vi "Convert_Message_For_Signal_Processing.vi"(1 "String":string) -> (0 "Array":i16[](array[numeric]))   [LabVIEW 2024]
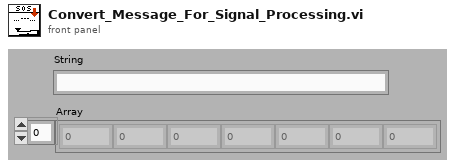
[diagram p1: front panel]
types:
  T1 = cluster{"0":bool[], "2":bool[], "4":bool[], "5":bool[], "6":bool[], "8":bool[], "9":bool[], "B":bool[], "C":bool[], "A":bool[], "D":bool[], "E":bool[], "7":bool[], "3":bool[], "1":bool[], "F":bool[], "G":bool[], "H":bool[], "I":bool[], "J":bool[], "K":bool[], "L":bool[], "M":bool[], "N":bool[], "O":bool[], "P":bool[], "Q":bool[], "R":bool[], "S":bool[], "T":bool[], "U":bool[], "V":bool[], "W":bool[], "X":bool[], "Y":bool[], "Z":bool[], ".":bool[], "?":bool[], ",":bool[], "/":bool[], "Space":bool[], "Null":bool[]}
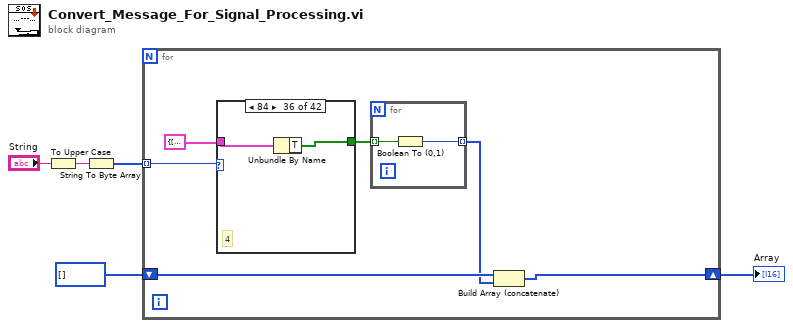
[diagram p0: block diagram]
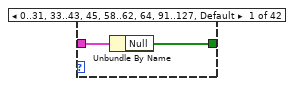
[diagram p2: hidden frame]
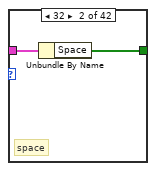
[diagram p3: hidden frame]
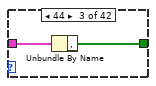
[diagram p4: hidden frame]
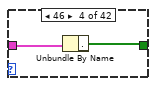
[diagram p5: hidden frame]
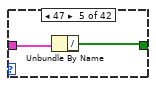
[diagram p6: hidden frame]
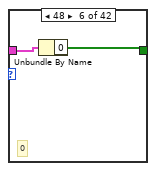
[diagram p7: hidden frame]
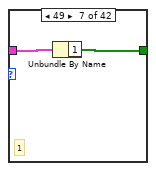
[diagram p8: hidden frame]
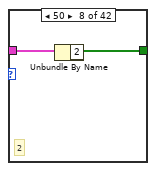
[diagram p9: hidden frame]
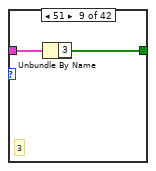
[diagram p10: hidden frame]
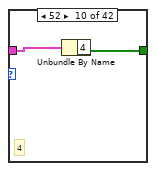
[diagram p11: hidden frame]
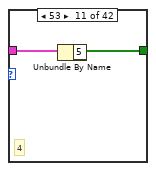
[diagram p12: hidden frame]
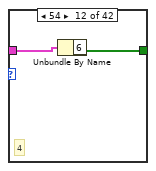
[diagram p13: hidden frame]
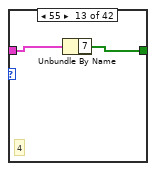
[diagram p14: hidden frame]
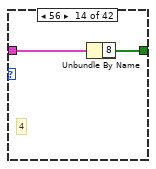
[diagram p15: hidden frame]
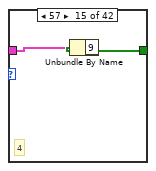
[diagram p16: hidden frame]
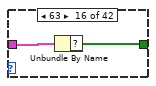
[diagram p17: hidden frame]
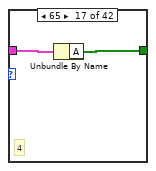
[diagram p18: hidden frame]
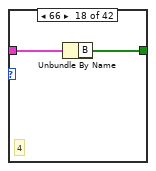
[diagram p19: hidden frame]
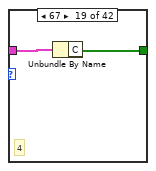
[diagram p20: hidden frame]
diagram:
  n1 = To Upper Case(1:"String") -> (0:w3:string)
  n2 = String To Byte Array(string=w3) -> (unsigned byte array=w4:u8[])
  n3 = for {
    tunnel: w4 -> [w10] mode=indexing
    shift-right: [w11] -> w1
    shift-left: i16[] [] -> [w9]
    n4 = case shown="84" w10 {
      tunnel: [w15 w17 w18 w20 w22 w25 w27 w29 w31 w33 w35 w37 w39 w41 w43 w45 w47 w49 w51 w53 w55 w57 w59 w61 w63 w65 w67 w69 w71 w73 w75 w77 w79 w81 w83 w85 w87 w89 w91 w92 w95 w97] -> w7
      tunnel: T1 {"0"=[TRUE, TRUE, TRUE, FALSE, TRUE, TRUE, TRUE, FALSE, TRUE, TRUE, TRUE, FALSE, TRUE, TRUE, TRUE, FALSE, TRUE, TRUE, TRUE, FALSE, FALSE, FALSE, FALSE, FALSE], "2"=[TRUE, FALSE, TRUE, FALSE, TRUE, TRUE, TRUE, FALSE, TRUE, TRUE, TRUE, FALSE, TRUE, TRUE, TRUE, FALSE, FALSE, FALSE, FALSE, FALSE], "4"=[TRUE, FALSE, TRUE, FALSE, TRUE, FALSE, TRUE, FALSE, TRUE, TRUE, TRUE, FALSE, FALSE, FALSE, FALSE, FALSE], "5"=[TRUE, FALSE, TRUE, FALSE, TRUE, FALSE, TRUE, FALSE, TRUE, FALSE, FALSE, FALSE, FALSE, FALSE], "6"=[TRUE, TRUE, TRUE, FALSE, TRUE, FALSE, TRUE, FALSE, TRUE, FALSE, TRUE, FALSE, FALSE, FALSE, FALSE, FALSE], "8"=[TRUE, TRUE, TRUE, FALSE, TRUE, TRUE, TRUE, FALSE, TRUE, TRUE, TRUE, FALSE, TRUE, FALSE, TRUE, FALSE, FALSE, FALSE, FALSE, FALSE], "9"=[TRUE, TRUE, TRUE, FALSE, TRUE, TRUE, TRUE, FALSE, TRUE, TRUE, TRUE, FALSE, TRUE, TRUE, TRUE, FALSE, TRUE, FALSE, FALSE, FALSE, FALSE, FALSE], "B"=[TRUE, TRUE, TRUE, FALSE, TRUE, FALSE, TRUE, FALSE, TRUE, FALSE, FALSE, FALSE, FALSE, FALSE], "C"=[TRUE, TRUE, TRUE, FALSE, TRUE, FALSE, TRUE, TRUE, TRUE, FALSE, TRUE, FALSE, FALSE, FALSE, FALSE, FALSE], "A"=[TRUE, FALSE, TRUE, TRUE, TRUE, FALSE, FALSE, FALSE, FALSE, FALSE], "D"=[TRUE, TRUE, TRUE, FALSE, TRUE, FALSE, TRUE, FALSE, FALSE, FALSE, FALSE, FALSE], "E"=[TRUE, FALSE, FALSE, FALSE, FALSE, FALSE], "7"=[TRUE, TRUE, TRUE, FALSE, TRUE, TRUE, TRUE, FALSE, TRUE, FALSE, TRUE, FALSE, TRUE, FALSE, FALSE, FALSE, FALSE, FALSE], "3"=[TRUE, FALSE, TRUE, FALSE, TRUE, FALSE, TRUE, TRUE, TRUE, FALSE, TRUE, TRUE, TRUE, FALSE, FALSE, FALSE, FALSE, FALSE], "1"=[TRUE, FALSE, TRUE, TRUE, TRUE, FALSE, TRUE, TRUE, TRUE, FALSE, TRUE, TRUE, TRUE, FALSE, TRUE, TRUE, TRUE, FALSE, FALSE, FALSE, FALSE, FALSE], "F"=[TRUE, FALSE, TRUE, FALSE, TRUE, TRUE, TRUE, FALSE, TRUE, FALSE, FALSE, FALSE, FALSE, FALSE], "G"=[TRUE, TRUE, TRUE, FALSE, TRUE, TRUE, TRUE, FALSE, TRUE, FALSE, FALSE, FALSE, FALSE, FALSE], "H"=[TRUE, FALSE, TRUE, FALSE, TRUE, FALSE, TRUE, FALSE, FALSE, FALSE, FALSE, FALSE], "I"=[TRUE, FALSE, TRUE, FALSE, FALSE, FALSE, FALSE, FALSE], "J"=[TRUE, FALSE, TRUE, TRUE, TRUE, FALSE, TRUE, TRUE, TRUE, FALSE, TRUE, TRUE, TRUE, FALSE, FALSE, FALSE, FALSE, FALSE], "K"=[TRUE, TRUE, TRUE, FALSE, TRUE, FALSE, TRUE, TRUE, TRUE, FALSE, FALSE, FALSE, FALSE, FALSE], "L"=[TRUE, FALSE, TRUE, TRUE, TRUE, FALSE, TRUE, FALSE, TRUE, FALSE, FALSE, FALSE, FALSE, FALSE], "M"=[TRUE, TRUE, TRUE, FALSE, TRUE, TRUE, TRUE, FALSE, FALSE, FALSE, FALSE, FALSE], "N"=[TRUE, TRUE, TRUE, FALSE, TRUE, FALSE, FALSE, FALSE, FALSE, FALSE], "O"=[TRUE, TRUE, TRUE, FALSE, TRUE, TRUE, TRUE, FALSE, TRUE, TRUE, TRUE, FALSE, FALSE, FALSE, FALSE, FALSE], "P"=[TRUE, FALSE, TRUE, TRUE, TRUE, FALSE, TRUE, TRUE, TRUE, FALSE, TRUE, FALSE, FALSE, FALSE, FALSE, FALSE], "Q"=[TRUE, TRUE, TRUE, FALSE, TRUE, TRUE, TRUE, FALSE, TRUE, FALSE, TRUE, TRUE, TRUE, FALSE, FALSE, FALSE, FALSE, FALSE], "R"=[TRUE, FALSE, TRUE, TRUE, TRUE, FALSE, TRUE, FALSE, FALSE, FALSE, FALSE, FALSE], "S"=[TRUE, FALSE, TRUE, FALSE, TRUE, FALSE, FALSE, FALSE, FALSE, FALSE], "T"=[TRUE, TRUE, TRUE, FALSE, FALSE, FALSE, FALSE, FALSE], "U"=[TRUE, FALSE, TRUE, FALSE, TRUE, TRUE, TRUE, FALSE, FALSE, FALSE, FALSE, FALSE], "V"=[TRUE, FALSE, TRUE, FALSE, TRUE, FALSE, TRUE, TRUE, TRUE, FALSE, FALSE, FALSE, FALSE, FALSE], "W"=[TRUE, FALSE, TRUE, TRUE, TRUE, FALSE, TRUE, TRUE, TRUE, FALSE, FALSE, FALSE, FALSE, FALSE], "X"=[TRUE, TRUE, TRUE, FALSE, TRUE, FALSE, TRUE, FALSE, TRUE, TRUE, TRUE, FALSE, FALSE, FALSE, FALSE, FALSE], "Y"=[TRUE, TRUE, TRUE, FALSE, TRUE, FALSE, TRUE, TRUE, TRUE, FALSE, TRUE, TRUE, TRUE, FALSE, FALSE, FALSE, FALSE, FALSE], "Z"=[TRUE, TRUE, TRUE, FALSE, TRUE, TRUE, TRUE, FALSE, TRUE, FALSE, TRUE, FALSE, FALSE, FALSE, FALSE, FALSE], "."=[TRUE, FALSE, TRUE, TRUE, TRUE, FALSE, TRUE, FALSE, TRUE, TRUE, TRUE, FALSE, TRUE, FALSE, TRUE, TRUE, TRUE, FALSE, FALSE, FALSE, FALSE, FALSE], "?"=[TRUE, FALSE, TRUE, FALSE, TRUE, TRUE, TRUE, FALSE, TRUE, TRUE, TRUE, FALSE, TRUE, FALSE, TRUE, FALSE, FALSE, FALSE, FALSE, FALSE], ","=[TRUE, TRUE, TRUE, FALSE, TRUE, TRUE, TRUE, FALSE, TRUE, FALSE, TRUE, FALSE, TRUE, TRUE, TRUE, FALSE, TRUE, TRUE, TRUE, FALSE, FALSE, FALSE, FALSE, FALSE], "/"=[TRUE, TRUE, TRUE, FALSE, TRUE, FALSE, TRUE, FALSE, TRUE, TRUE, TRUE, FALSE, TRUE, FALSE, FALSE, FALSE, FALSE, FALSE], "Space"=[FALSE, FALSE, FALSE, FALSE, FALSE, FALSE, FALSE], "Null"=[]} -> [w14 w16 w19 w21 w23 w24 w26 w28 w30 w32 w34 w36 w38 w40 w42 w44 w46 w48 w50 w52 w54 w56 w58 w60 w62 w64 w66 w68 w70 w72 w74 w76 w78 w80 w82 w84 w86 w88 w90 w93 w94 w96]
      frame 0..31, 33..43, 45, 58..62, 64, 91..127, Default {
        n5 = Unbundle By Name(w14) -> ("Null"=w15:bool[])
      }
      frame 32 {
        # "space"
        n6 = Unbundle By Name(w16) -> ("Space"=w17:bool[])
      }
      frame 44 {
        n7 = Unbundle By Name(w19) -> (","=w18:bool[])
      }
      frame 46 {
        n8 = Unbundle By Name(w21) -> ("."=w20:bool[])
      }
      frame 47 {
        n9 = Unbundle By Name(w23) -> ("/"=w22:bool[])
      }
      frame 48 {
        # "0"
        n10 = Unbundle By Name(w24) -> ("0"=w25:bool[])
      }
      frame 49 {
        # "1"
        n11 = Unbundle By Name(w26) -> ("1"=w27:bool[])
      }
      frame 50 {
        # "2"
        n12 = Unbundle By Name(w28) -> ("2"=w29:bool[])
      }
      frame 51 {
        # "3"
        n13 = Unbundle By Name(w30) -> ("3"=w31:bool[])
      }
      frame 52 {
        # "4"
        n14 = Unbundle By Name(w32) -> ("4"=w33:bool[])
      }
      frame 53 {
        # "4"
        n15 = Unbundle By Name(w34) -> ("5"=w35:bool[])
      }
      frame 54 {
        # "4"
        n16 = Unbundle By Name(w36) -> ("6"=w37:bool[])
      }
      frame 55 {
        # "4"
        n17 = Unbundle By Name(w38) -> ("7"=w39:bool[])
      }
      frame 56 {
        # "4"
        n18 = Unbundle By Name(w40) -> ("8"=w41:bool[])
      }
      frame 57 {
        # "4"
        n19 = Unbundle By Name(w42) -> ("9"=w43:bool[])
      }
      frame 63 {
        n20 = Unbundle By Name(w44) -> ("?"=w45:bool[])
      }
      frame 65 {
        # "4"
        n21 = Unbundle By Name(w46) -> ("A"=w47:bool[])
      }
      frame 66 {
        # "4"
        n22 = Unbundle By Name(w48) -> ("B"=w49:bool[])
      }
      frame 67 {
        # "4"
        n23 = Unbundle By Name(w50) -> ("C"=w51:bool[])
      }
      frame 68 {
        # "4"
        n24 = Unbundle By Name(w52) -> ("D"=w53:bool[])
      }
      frame 69 {
        # "4"
        n25 = Unbundle By Name(w54) -> ("E"=w55:bool[])
      }
      frame 70 {
        # "4"
        n26 = Unbundle By Name(w56) -> ("F"=w57:bool[])
      }
      frame 71 {
        # "4"
        n27 = Unbundle By Name(w58) -> ("G"=w59:bool[])
      }
      frame 72 {
        # "4"
        n28 = Unbundle By Name(w60) -> ("H"=w61:bool[])
      }
      frame 73 {
        # "4"
        n29 = Unbundle By Name(w62) -> ("I"=w63:bool[])
      }
      frame 74 {
        # "4"
        n30 = Unbundle By Name(w64) -> ("J"=w65:bool[])
      }
      frame 75 {
        # "4"
        n31 = Unbundle By Name(w66) -> ("K"=w67:bool[])
      }
      frame 76 {
        # "4"
        n32 = Unbundle By Name(w68) -> ("L"=w69:bool[])
      }
      frame 77 {
        # "4"
        n33 = Unbundle By Name(w70) -> ("M"=w71:bool[])
      }
      frame 78 {
        # "4"
        n34 = Unbundle By Name(w72) -> ("N"=w73:bool[])
      }
      frame 79 {
        # "4"
        n35 = Unbundle By Name(w74) -> ("O"=w75:bool[])
      }
      frame 80 {
        # "4"
        n36 = Unbundle By Name(w76) -> ("P"=w77:bool[])
      }
      frame 81 {
        # "4"
        n37 = Unbundle By Name(w78) -> ("Q"=w79:bool[])
      }
      frame 82 {
        # "4"
        n38 = Unbundle By Name(w80) -> ("R"=w81:bool[])
      }
      frame 83 {
        # "4"
        n39 = Unbundle By Name(w82) -> ("S"=w83:bool[])
      }
      frame 84 {
        # "4"
        n40 = Unbundle By Name(w84) -> ("T"=w85:bool[])
      }
      frame 85 {
        # "4"
        n41 = Unbundle By Name(w86) -> ("U"=w87:bool[])
      }
      frame 86 {
        # "4"
        n42 = Unbundle By Name(w88) -> ("V"=w89:bool[])
      }
      frame 87 {
        # "4"
        n43 = Unbundle By Name(w90) -> ("W"=w91:bool[])
      }
      frame 88 {
        # "4"
        n44 = Unbundle By Name(w93) -> ("X"=w92:bool[])
      }
      frame 89 {
        # "4"
        n45 = Unbundle By Name(w94) -> ("Y"=w95:bool[])
      }
      frame 90 {
        # "4"
        n46 = Unbundle By Name(w96) -> ("Z"=w97:bool[])
      }
    }
    n47 = for {
      tunnel: w7 -> [w12] mode=indexing
      tunnel: [w13] -> w6 mode=indexing
      n48 = Boolean To (0,1)(Boolean=w12) -> (0, 1=w13:i16)
    }
    n49 = Build Array (concatenate)(w9, w6) -> (w11:i16[])
  }
  "Array" <- w1
